vi "ad get range count.vi"(8 "error in (no error)":errorcluster, 9 "cnt":i32, 10 "cha":i32, 11 "adh":i32) -> (0 "error out":errorcluster, 3 "function return":i32)   [LabVIEW 2021, in "libad4.lvlib"]
doc: "LIBAD4 function: ad_get_range_count (int32_t adh, int32_t cha, int32_t *cnt);\n\nReturns the number of measuring ranges of the channel `cha`."
uses:
  <userlib>/libad4/libad4.lvlib
  <userlib>/libad4/libad4.dll
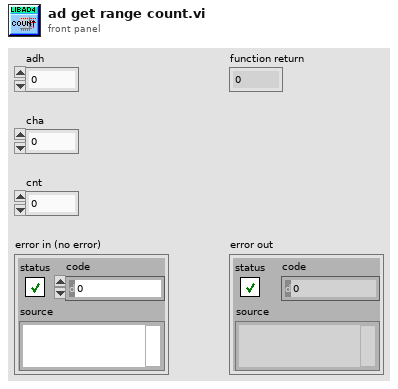
[diagram p1: front panel]
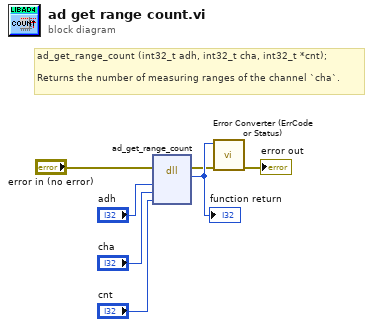
[diagram p0: block diagram]
diagram:
  # "ad_get_range_count (int32_t adh, int32_t cha, int32_t *cnt);\n\nReturns the number of measuring ranges of the channel `cha`."
  n1 = dll-call lib="C:/Program Files/National Instruments/LabVIEW 2021/user.lib/libad4/libad4.*" fn="ad_get_range_count"(error in="error in (no error)", "adh"="adh", "cha"="cha", "cnt"="cnt") -> (error out=w2:errorcluster, "return type"=w7:i32)  [unwired: 5 in, 1 out]
  "function return" <- w7
  n2 = call <userlib>:"Error Converter (ErrCode or Status).vi"("error in (no error)"=w2, "error code"=w7) -> ("error out"=→"error out":errorcluster)  [unwired: 9 in]
